vi "serialize_test.vi"() -> ()   [LabVIEW 2019]
uses:
  5236ca62-83be-4ce2-a2f0-a16833f629fd.vi
  e6657b15-3961-4f78-acc7-f12dbd3bd8cd.vi
  <vilib>/JDP Science/JSONtext/Variant to JSON Text.vi
  <vilib>/JDP Science/JSONtext/JSON text to Variant.vi
  <vilib>/JDP Science/JSONtext/LVClass Serializer/JSONtext LVClass Serializer.lvclass
  <vilib>/addons/_JKI.lib/Serialization/JSON/JKI JSON Serialization.lvlib
  <vilib>/measure/NI_MABase.lvlib
panel:
  out "X to data?":bool
  out "data to X?":bool
  in  "X":enum16{"JSON", "JSONtext", "Flatten"}(ring)
  out "X to data":dbl format="%#_6p"
  out "data to X":dbl format="%#_6p"
  out "data":waveform(dbl)[](array[waveform])
  out "input signal":waveform(dbl)[](array[waveform])
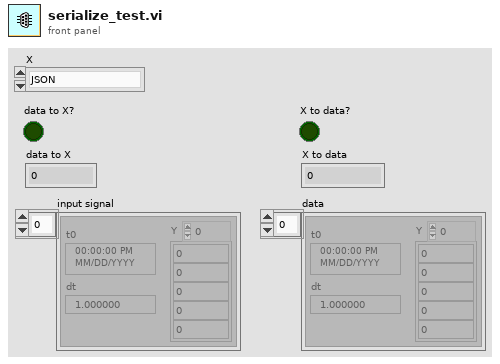
[diagram p1: front panel]
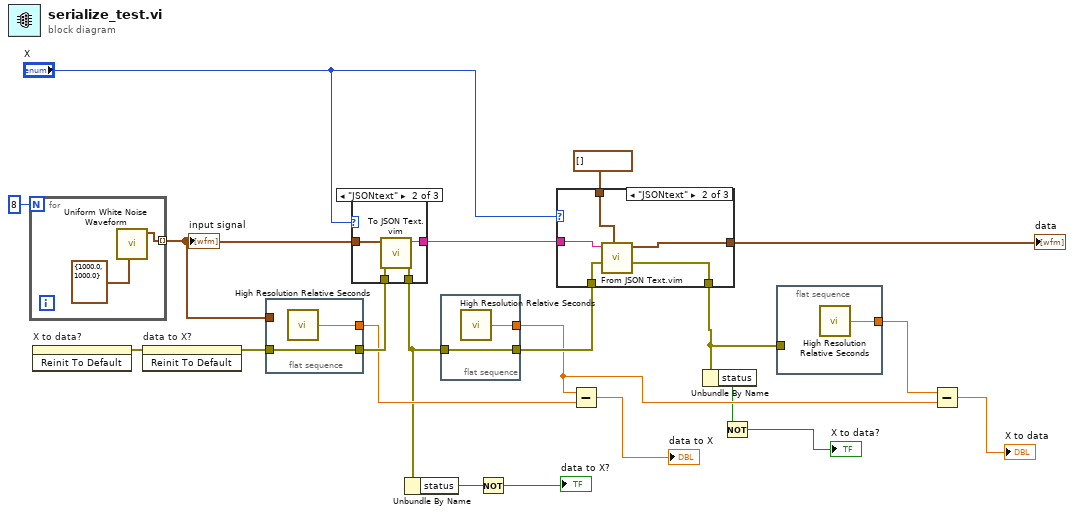
[diagram p0: block diagram]
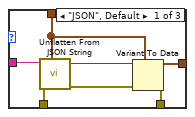
[diagram p2: hidden frame]
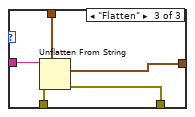
[diagram p3: hidden frame]
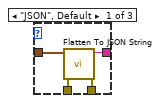
[diagram p4: hidden frame]
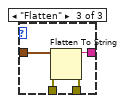
[diagram p5: hidden frame]
diagram:
  n1 = for {
    N: 8 -> [_]
    tunnel: [w22] -> w1 mode=indexing
    n2 = call <vilib>:"Uniform White Noise Waveform.vi"("sampling info"=cluster{"Fs":dbl, "#s":dbl} {"Fs"=1000.0, "#s"=1000.0}) -> ("signal out"=w22:waveform(dbl))  [unwired: 9 in, 1 out]
  }
  "input signal" <- w1
  n3 = invoke on="X to data?" class="Bool (strict)" method="Reinit To Default"() -> (error out=w6:errorcluster)  [unwired: 3 in, 2 out]
  n4 = invoke on="data to X?" class="Bool (strict)" method="Reinit To Default"(error in=w6) -> (error out=w5:errorcluster)  [unwired: 2 in, 2 out]
  n5 = flat-sequence {
    tunnel: [w24] -> w19
    tunnel: [w25] -> w17
    tunnel: w5 -> [w24]
    tunnel: w1 -> [_]
    frame #0 {
      n6 = call <vilib>:"High Resolution Relative Seconds.vi"() -> ("relative seconds"=w25:dbl)
    }
  }
  n7 = case shown="\"JSONtext\"" "X" {
    tunnel: [w29 w30 w36] -> w21
    tunnel: [w28 w31 w34] -> w10
    tunnel: w19 -> [w27 w32 w35]
    tunnel: w1 -> [w26 w33 w37]
    frame "JSON", Default {
      n8 = call <vilib>:"Flatten To JSON String.vi"("error in (no error)"=w27, "Variant"=w26) -> ("error out"=w28:errorcluster, "JSON String"=w29:string)  [unwired: 8 in]
    }
    frame "JSONtext" {
      n9 = call "To JSON Text.vim"("error in (no error)"=w32, "Anything"=w33) -> ("error out"=w31:errorcluster, "<JSON>"=w30:string)  [unwired: 8 in]
    }
    frame "Flatten" {
      n10 = Flatten To String(anything=w37, error in (no error)=w35) -> (data string=w36:string, error out=w34:errorcluster)  [unwired: 2 in, 1 out]
    }
  }
  n11 = Unbundle By Name(w10) -> ("status"=w9:bool)
  n12 = flat-sequence {
    tunnel: [w38] -> w18
    tunnel: [w39] -> w13
    tunnel: w10 -> [w38]
    frame #0 {
      n13 = call <vilib>:"High Resolution Relative Seconds.vi"() -> ("relative seconds"=w39:dbl)
    }
  }
  n14 = Not(x=w9) -> (.not. x?=→"data to X?":bool)
  n15 = case shown="\"JSONtext\"" "X" {
    tunnel: w21 -> [w46 w50 w56]
    tunnel: [w44 w47 w53] -> w20
    tunnel: [w42 w48 w52] -> w8
    tunnel: w18 -> [w41 w49 w55]
    tunnel: waveform(dbl)[] [] ("input signal 2") -> [w40 w51 w54]
    frame "JSON", Default {
      n16 = call <vilib>:"Unflatten From JSON String.vi"("Type and Defaults"=w40, "error in (no error)"=w41, "JSON String"=w46) -> ("error out"=w43:errorcluster, "Variant"=w45:variant)  [unwired: 7 in]
      n17 = Variant To Data(error in=w43, type=w40, Variant=w45) -> (data=w44:waveform(dbl)[], error out=w42:errorcluster)
    }
    frame "JSONtext" {
      n18 = call "From JSON Text.vim"("Data Type and Default Value"=w51, "error in (no error)"=w49, "JSON"=w50) -> ("error out"=w48:errorcluster, "Data out"=w47:waveform(dbl)[])  [unwired: 7 in]
    }
    frame "Flatten" {
      n19 = Unflatten From String(type=w54, binary string=w56, error in (no error)=w55) -> (value=w53:waveform(dbl)[], error out=w52:errorcluster)  [unwired: 2 in, 1 out]
    }
  }
  "data" <- w20
  n20 = Subtract(x=w13, y=w17) -> (x-y=→"data to X":dbl)
  n21 = Unbundle By Name(w8) -> ("status"=w7:bool)
  n22 = Not(x=w7) -> (.not. x?=→"X to data?":bool)
  n23 = flat-sequence {
    tunnel: [w57] -> w16
    tunnel: w8 -> [_]
    frame #0 {
      n24 = call <vilib>:"High Resolution Relative Seconds.vi"() -> ("relative seconds"=w57:dbl)
    }
  }
  n25 = Subtract(x=w16, y=w13) -> (x-y=→"X to data":dbl)
